vi "toml.create.vi"(8 "error in":errorcluster, 11 "configuration-data":refnum<class "configuration-data.lvclass">) -> (0 "error out":errorcluster, 3 "toml":string)   [LabVIEW 2020, in "configuration-data.lvclass"]
uses:
  configuration-data.lvclass
  configuration-data.lvclass/configuration-data.ctl
  4f0fa088-b6c6-485f-af08-1b988c6e672f.vi
  6526c327-a351-431d-8d48-74aed546e54b.vi
  255e6a50-431b-42dd-aa7d-2e2d022d1bd1.vi
  276128d2-df76-4891-9c63-49da039d568e.vi
  4f0fa088-b6c6-485f-af08-1b988c6e672f.vi/4178f046-9af6-4db4-9405-99552d650b27.vi
  4f0fa088-b6c6-485f-af08-1b988c6e672f.vi/504846f3-46c1-483c-ab2c-e4b1da560c38.vi
  6526c327-a351-431d-8d48-74aed546e54b.vi/4178f046-9af6-4db4-9405-99552d650b27.vi
  6526c327-a351-431d-8d48-74aed546e54b.vi/504846f3-46c1-483c-ab2c-e4b1da560c38.vi
  255e6a50-431b-42dd-aa7d-2e2d022d1bd1.vi/4178f046-9af6-4db4-9405-99552d650b27.vi
  255e6a50-431b-42dd-aa7d-2e2d022d1bd1.vi/504846f3-46c1-483c-ab2c-e4b1da560c38.vi
  255e6a50-431b-42dd-aa7d-2e2d022d1bd1.vi/59a7dd5e-ca60-4e8a-acbf-a4720f172a4c.vi
  276128d2-df76-4891-9c63-49da039d568e.vi/4178f046-9af6-4db4-9405-99552d650b27.vi
  276128d2-df76-4891-9c63-49da039d568e.vi/504846f3-46c1-483c-ab2c-e4b1da560c38.vi
  Item/from_boolean.vi
  toml/write_subtable_key_string.vi
  Item/from_integer.vi
  toml/toml.lvclass
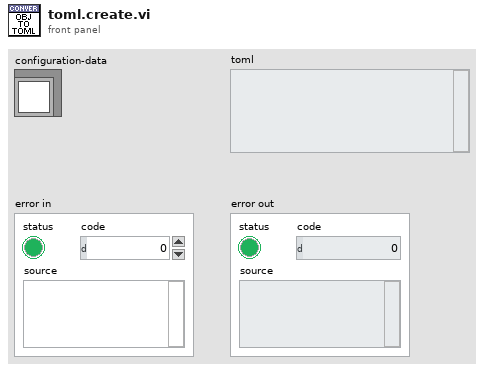
[diagram p1: front panel]
types:
  T1 = typedef "configuration-data.lvclass/configuration--map.ctl" = map{string, map{string, T2}}
  T2 = typedef "configuration-data.lvclass/value--cluster.ctl" = cluster{"datatype":T3, "value":variant}
  T3 = typedef "configuration-data.lvclass/datatype--enum.ctl" = enum16{"Boolean", "Double", "Integer", "String"}
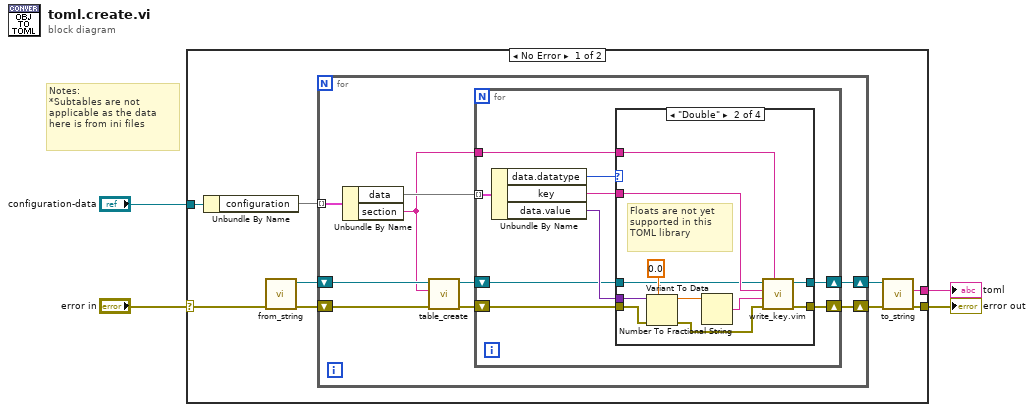
[diagram p0: block diagram]
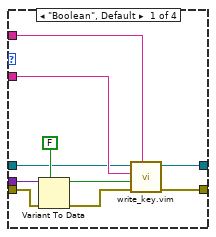
[diagram p2: hidden frame]
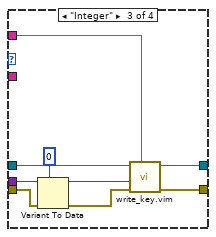
[diagram p3: hidden frame]
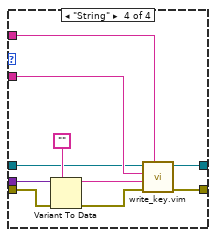
[diagram p4: hidden frame]
diagram:
  # "Notes:\n*Subtables are not applicable as the data here is from ini files"
  n1 = case shown="No Error" "error in" {
    selector: "error in" -> [w12 w72]
    tunnel: "configuration-data" -> [w13 _]
    tunnel: [w8 _] -> w2
    tunnel: [w6 w72] -> w1
    frame No Error {
      n2 = Unbundle By Name(w13) -> ("configuration"=w10:T1)
      n3 = call "from_string.vi"("error in (no error)"=w12) -> ("error out"=w11:errorcluster, "toml out"=w9:refnum<class "toml.lvclass">)  [unwired: 9 in]
      n4 = for {
        tunnel: w10 -> [w22] mode=indexing
        shift-right: [w15] -> w7
        shift-left: w9 -> [w20]
        shift-right: [w14] -> w5
        shift-left: w11 -> [w19]
        n5 = Unbundle By Name(w22) -> ("data"=w21:map{string, T2}, "section"=w17:string)
        n6 = call "table_create.vi"("error in (no error)"=w19, "table name"=w17, "toml in"=w20) -> ("error out"=w16:errorcluster, "toml out"=w18:refnum<class "toml.lvclass">)  [unwired: 6 in, 1 out]
        n7 = for {
          tunnel: w21 -> [w31] mode=indexing
          shift-right: [w26] -> w15
          shift-left: w18 -> [w25]
          tunnel: w17 -> [w29]
          shift-right: [w24] -> w14
          shift-left: w16 -> [w27]
          n8 = Unbundle By Name(w31) -> ("data.datatype"=w23:T3, "key"=w30:string, "data.value"=w28:variant)
          n9 = case shown="\"Double\"" w23 {
            tunnel: w30 -> [w38 w51 _ w67]
            tunnel: w29 -> [w39 w52 w58 w66]
            tunnel: w28 -> [w37 w49 w59 w70]
            tunnel: w27 -> [w35 w47 w54 w64]
            tunnel: [w34 w45 w55 w63] -> w26
            tunnel: w25 -> [w33 w46 w56 w65]
            tunnel: [w32 w42 w53 w62] -> w24
            frame "Boolean", Default {
              n10 = Variant To Data(error in=w35, type=FALSE, Variant=w37) -> (data=w41:bool, error out=w36:errorcluster)
              n11 = call "write_key.vim"("table"=w39, "error in (no error)"=w36, "value"=w41, "key"=w38, "toml in"=w33) -> ("error out"=w32:errorcluster, "toml out"=w34:refnum<class "toml.lvclass">)  [unwired: 5 in]
            }
            frame "Double" {
              # "Floats are not yet supported in this TOML library"
              n12 = Variant To Data(error in=w47, type=0.0 ("double precision float"), Variant=w49) -> (data=w44:dbl, error out=w50:errorcluster)
              n13 = Number To Fractional String(number=w44) -> (F-format string=w43:string)  [unwired: 3 in]
              n14 = call "write_key.vim"("table"=w52, "error in (no error)"=w50, "value"=w43, "key"=w51, "toml in"=w46) -> ("error out"=w42:errorcluster, "toml out"=w45:refnum<class "toml.lvclass">)  [unwired: 5 in]
            }
            frame "Integer" {
              n15 = Variant To Data(error in=w54, type=i64 0, Variant=w59) -> (data=w60:i64, error out=w61:errorcluster)
              n16 = call "write_key.vim"("table"=w58, "error in (no error)"=w61, "value"=w60, "toml in"=w56) -> ("error out"=w53:errorcluster, "toml out"=w55:refnum<class "toml.lvclass">)  [unwired: 6 in]
            }
            frame "String" {
              n17 = Variant To Data(error in=w64, type="", Variant=w70) -> (data=w71:string, error out=w69:errorcluster)
              n18 = call "write_key.vim"("table"=w66, "error in (no error)"=w69, "value"=w71, "key"=w67, "toml in"=w65) -> ("error out"=w62:errorcluster, "toml out"=w63:refnum<class "toml.lvclass">)  [unwired: 5 in]
            }
          }
        }
      }
      n19 = call "to_string.vi"("error in (no error)"=w5, "toml in"=w7) -> ("error out"=w6:errorcluster, "toml_string"=w8:string)  [unwired: 8 in]
    }
    frame Error {
    }
  }
  "error out" <- w1
  "toml" <- w2
